vi "build path cluster.vi"() -> ()   [LabVIEW 2025, in "Motor.lvlib"]
uses:
  Path Mode.ctl
  Motor.lvlib
panel:
  in  "Cluster 2":T2
  out "Cluster":T2
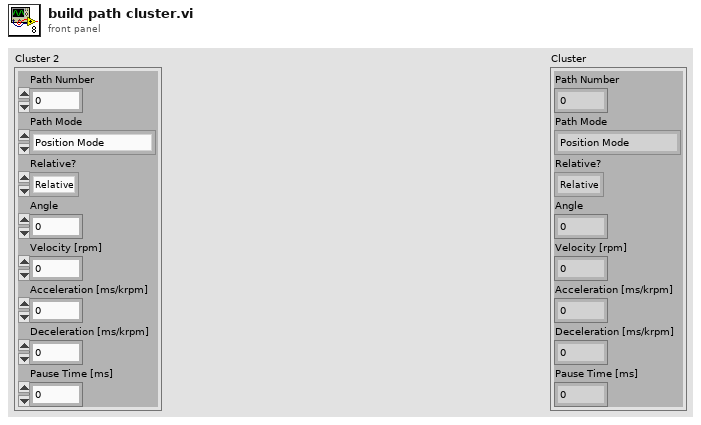
[diagram p1: front panel]
types:
  T1 = typedef "Motor.lvlib/Path Mode.ctl" = enum16{"Position Mode", "Velocity Mode", "Homing Mode"}
  T2 = cluster{"Path Number":i32, "Path Mode":T1, "Relative?":enum16{"Relative", "Absolute"}, "Angle":dbl, "Velocity [rpm]":i32, "Acceleration [ms/krpm]":i32, "Deceleration [ms/krpm]":i32, "Pause Time [ms]":i32}
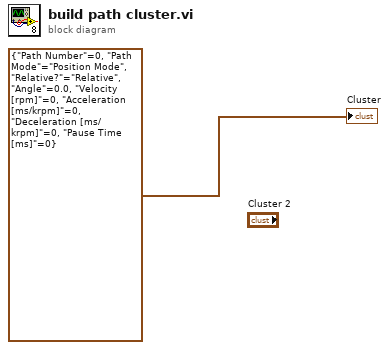
[diagram p0: block diagram]
diagram:
  "Cluster" <- T2 {"Path Number"=0, "Path Mode"=enum."Position Mode", "Relative?"=enum."Relative", "Angle"=0.0, "Velocity [rpm]"=0, "Acceleration [ms/krpm]"=0, "Deceleration [ms/krpm]"=0, "Pause Time [ms]"=0}
